vi "Host Run 5 Wire xVDT Sim.vi"() -> ()   [LabVIEW 2011]
uses:
  <vilib>/rvi/interface/nirviCloseFPGA/nirviCloseFPGA.xnode
  <vilib>/rvi/interface/nirviOpenFPGA/nirviOpenFPGA.xnode
  <vilib>/rvi/interface/nirviReadWriteControl/nirviReadWriteControl.xnode
  FPGA/FPGA 5 Wire xVDT Sim.vi
  FPGA Bitfiles/xVDTSimulation_7852_FPGA5WirexVDTSim_E80FE297.lvbitx
  <vilib>/FPGAPlugInAG/PXI-7852R/niLvFpga_Open_PXI-7852R.vi
  <vilib>/rvi/errors/niLvFpgaMergeErrorWithErrorCode.vi
  <vilib>/rvi/errors/niLvFpgaAdjustHostInterfaceError.vi
  <vilib>/FPGAPlugInAG/PXI-7852R/niLvFpga_Close_PXI-7852R.vi
panel:
  in  "Transfer ratio":dbl=0.6
  out "Scaling Factor 2":fxp<+/-,19,5> format="%.16g"
  out "Scaling Factor":fxp<+/-,19,5> format="%.16g"
  in  "Difference over sum gain":dbl=0.05
  out "error out":errorcluster
  in  "stop":bool
  in  "Position (mm)":dbl(slide) caption="Position" scale=-10.0..10.0 scale format="%.2f"
  # "Setup"
  # "Run-Time"
  # "Transfer Ratio or Sum Ratio = (Va+Vb)/Ve"
  # "Difference over sum gain = ((Va-Vb)/(Va+Vb))/d"
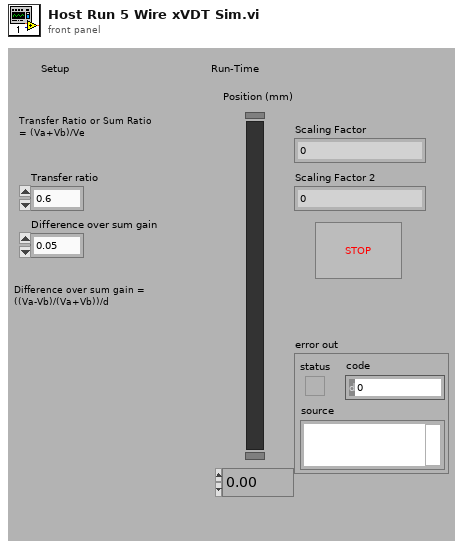
[diagram p1: front panel]
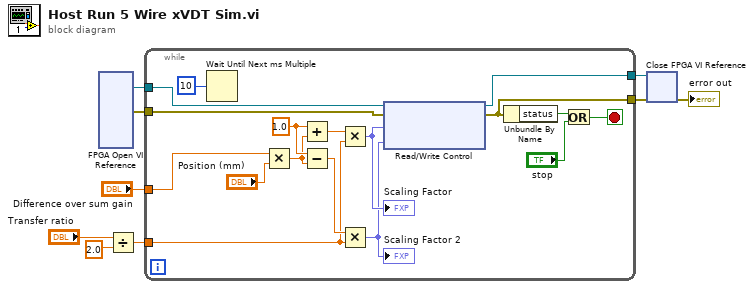
[diagram p0: block diagram]
diagram:
  n1 = xnode "FPGA Open VI Reference"() -> ("FPGA VI Reference Out"=w7:refnum<k20>, "error out"=w6:errorcluster)  [unwired: 2 in]
  n2 = Divide(x="Transfer ratio", y=2.0 ("x")) -> (x/y=w1:dbl)
  n3 = while {
    tunnel: w6 -> [w20]
    tunnel: [w22] -> w9
    tunnel: w7 -> [w21]
    tunnel: [w19] -> w5
    tunnel: "Difference over sum gain" -> [w17]
    tunnel: w1 -> [w13]
    stop <- w24 stop-if-true
    w16 = 1.0 ("x")
    n4 = Wait Until Next ms Multiple(millisecond multiple=u32 10) -> ()  [unwired: 1 out]
    n5 = Multiply(x=w17, y="Position (mm)") -> (x*y=w12:dbl)
    n6 = Add(x=w16, y=w12) -> (x+y=w15:dbl)
    n7 = Subtract(x=w16, y=w12) -> (x-y=w14:dbl)
    n8 = Multiply(x=w15, y=w13) -> (x*y=w11:fxp<+/-,19,5>)
    "Scaling Factor" <- w11
    n9 = Multiply(x=w14, y=w13) -> (x*y=w10:fxp<+/-,19,5>)
    "Scaling Factor 2" <- w10
    n10 = xnode "Read/Write Control"("FPGA VI Reference In"=w21, "error in"=w20, "Scaling Factor"=w11, "Scaling Factor 2"=w10) -> ("FPGA VI Reference Out"=w19:refnum<k20>, "error out"=w22:errorcluster)
    n11 = Unbundle By Name(w22) -> ("status"=w23:bool)
    n12 = Or(x=w23, y="stop") -> (x .or. y?=w24:bool)
  }
  n13 = xnode "Close FPGA VI Reference"("FPGA VI Reference In"=w5, "error in"=w9) -> ("error out"=→"error out":errorcluster)
